vi "coler1.vi"(8 "error in":errorcluster, 11 "代刚":bool) -> (0 "error out":errorcluster, 1 "顏色":enum16{"黑色", "藍色", "綠色", "黃色", "紅色"}[](array[ring]))   [LabVIEW 2018]
uses:
  <vilib>/vision/NI_Vision_Development_Module.lvlib
panel:
  out "5":u32(colorbox)
  out "4":u32(colorbox)
  out "3":u32(colorbox)
  out "2":u32(colorbox)
  out "1":u32(colorbox)
  out "Color":u32(colorbox)
  out "亮度":dbl[](array[numeric])
  out "︹办":dbl[](array[numeric])
  out "Image Out":T1(plugin-control)
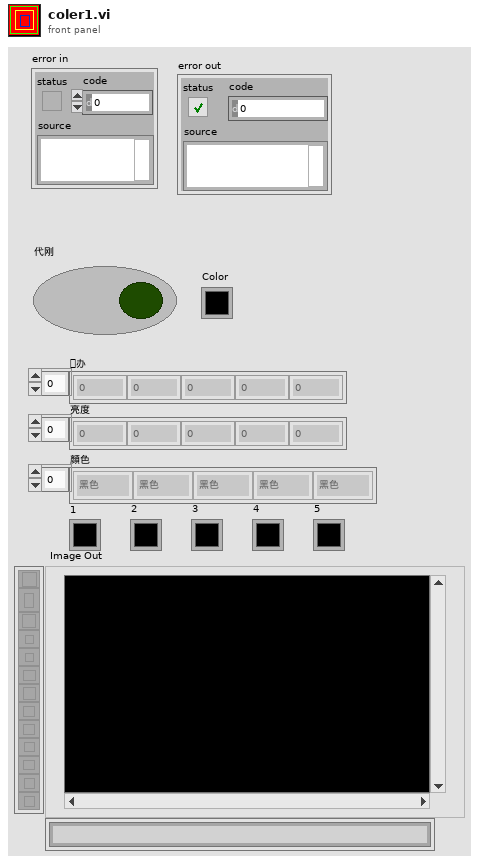
[diagram p1: front panel]
types:
  T1 = typedef "IMAQ Image.ctl" = refnum<image>
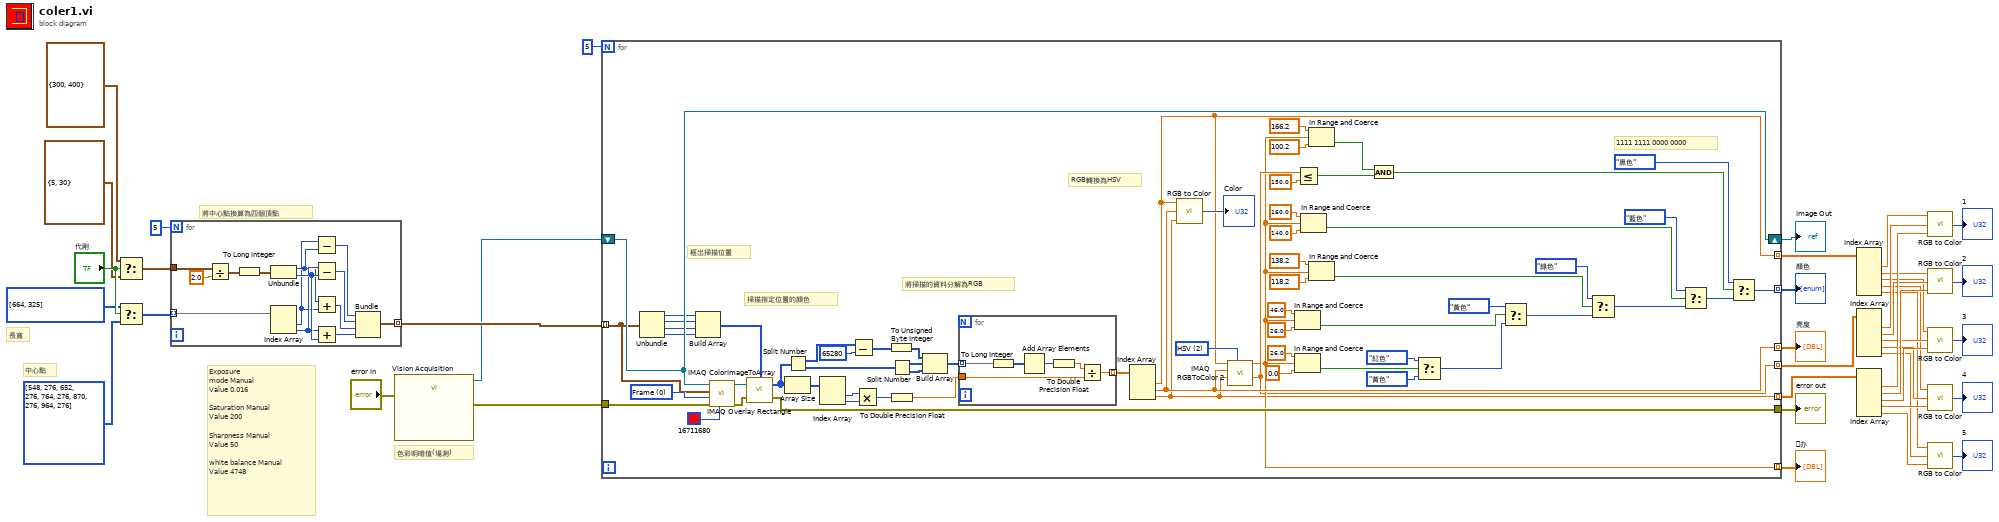
[diagram p0: block diagram]
diagram:
  # "長寬"
  # "Exposure\nmode Manual\nValue 0.016\n\nSaturation Manual\nValue 200\n\nSharpness Manual\nValue 50\n\nwhite balance Manual \nValue 4748"
  # "色彩明暗值(場測)"
  # "中心點"
  # "將中心點換算為四個頂點"
  n1 = Select(t=cluster{i32, i32} {300, 400}, s="代刚", f=cluster{i32, i32} {5, 30}) -> (s? t:f=w36:cluster{i32, i32})
  n2 = Select(t=i32[][] [[664, 325]], s="代刚", f=i32[][] [[548, 276], [652, 276], [764, 276], [870, 276], [964, 276]]) -> (s? t:f=w37:i32[][])
  n3 = for {
    N: 5 -> [_]
    tunnel: w36 -> [w55]
    tunnel: w37 -> [w52] mode=indexing
    tunnel: [w42] -> w38 mode=indexing
    n4 = Divide(x=w55, y=2.0) -> (x/y=w53:cluster{dbl, dbl})
    n5 = To Long Integer(number=w53) -> (32bit integer=w51:cluster{i32, i32})
    n6 = Unbundle(w51) -> (w48:i32, w50:i32)
    n7 = Index Array(array=w52) -> (element #1=w47:i32, element #2=w49:i32)  [unwired: 2 in]
    n8 = Subtract(x=w47, y=w48) -> (x-y=w46:i32)
    n9 = Subtract(x=w49, y=w50) -> (x-y=w45:i32)
    n10 = Add(x=w48, y=w47) -> (x+y=w44:i32)
    n11 = Add(x=w49, y=w50) -> (x+y=w43:i32)
    n12 = Bundle(w46, w45, w44, w43) -> (w42:cluster{i32, i32, i32, i32})  [unwired: 1 in]
  }
  n13 = call "Vision Acquisition"("error in"="error in") -> ("Image Out"=w33:T1, "error out"=w35:errorcluster)  [unwired: 25 in]
  n14 = for {
    N: 5 -> [_]
    shift-right: [w100] -> w34
    shift-left: w33 -> [w100]
    tunnel: w35 -> [w102]
    tunnel: [w101] -> w41
    tunnel: w38 -> [w96] mode=indexing
    tunnel: [w60] -> w26 mode=indexing
    tunnel: [w87] -> w25 mode=indexing
    tunnel: [w70] -> w24 mode=indexing
    tunnel: [w58] -> w23 mode=indexing
    tunnel: [w57] -> w22 mode=indexing
    tunnel: [w56] -> w21 mode=indexing
    w104 = u16 2 items=["RGB", "HSL", "HSV", "HSI", "CIE L*a*b*", "CIE XYZ"] ("Color Mode")
    w119 = u32 0 items=["Frame", "Fill", "Highlight"] ("Drawing Mode (Frame)")
    # "RGB轉換為HSV"
    # "將掃描的資料分解為RGB"
    # "掃描指定位置的顏色"
    # "框出掃描位置"
    # "1111 1111 0000 0000"
    n15 = Unbundle(w96) -> (w95:i32, w94:i32, w93:i32, w92:i32)
    n16 = Build Array(w95, w94, w93, w92) -> (w91:i32[])
    n17 = call "IMAQ Overlay Rectangle"("Color"=u32 16711680, "error in (no error)"=w102, "Drawing Mode (Frame)"=w119, "Rectangle"=w96, "Image"=w100) -> ("error out"=w98:errorcluster, "Image Out"=w99:T1)  [unwired: 5 in]
    n18 = call "IMAQ ColorImageToArray"("Optional Rectangle"=w91, "Image"=w99, "error in (no error)"=w98) -> ("Image Pixels (U32)"=w118:u32[][], "error out"=w101:errorcluster)  [unwired: 1 in, 1 out]
    n19 = Array Size(array=w118) -> (size(s)=w117:i32[])
    n20 = Split Number(x=w118) -> (hi(x)=w97:u16[][], lo(x)=w114:u16[][])
    n21 = Index Array(array=w117) -> (element #1=w108:i32, element #2=w109:i32)  [unwired: 2 in]
    n22 = Subtract(x=w97, y=u16 65280) -> (x-y=w115:u16[][])
    n23 = Multiply(x=w108, y=w109) -> (x*y=w107:i32)
    n24 = To Unsigned Byte Integer(number=w115) -> (unsigned 8bit integer=w113:u8[][])
    n25 = To Double Precision Float(number=w107) -> (double precision float=w106:dbl)
    n26 = Split Number(x=w114) -> (hi(x)=w112:u8[][], lo(x)=w111:u8[][])
    n27 = Build Array(w113, w112, w111) -> (w110:u8[][][])
    n28 = for {
      tunnel: w110 -> [w125] mode=indexing
      tunnel: w106 -> [w123]
      tunnel: [w122] -> w105 mode=indexing
      n29 = To Long Integer(number=w125) -> (32bit integer=w124:i32[][])
      n30 = Add Array Elements(numeric array=w124) -> (sum=w121:i32)
      n31 = To Double Precision Float(number=w121) -> (double precision float=w120:dbl)
      n32 = Divide(x=w120, y=w123) -> (x/y=w122:dbl)
    }
    n33 = Index Array(array=w105) -> (element #1=w58:dbl, element #2=w57:dbl, element #3=w56:dbl)  [unwired: 3 in]
    n34 = call <vilib>:"RGB to Color.vi"("B"=w56, "G"=w57, "R"=w58) -> ("Color"=→"Color":u32)
    n35 = call "IMAQ RGBToColor 2"("Color Mode"=w104, "Blue value"=w56, "Green value"=w57, "Red value"=w58) -> ("Blue or Luma or Val or Inten or Z or b*value"=w87:dbl, "Red or Hue or X or L* value"=w60:dbl)  [unwired: 4 in, 2 out]
    n36 = In Range and Coerce(upper limit=46.0, x=w60, lower limit=26.0) -> (In Range?=w72:bool)  [unwired: 1 out]
    n37 = In Range and Coerce(upper limit=26.0, x=w60, lower limit=0.0) -> (In Range?=w63:bool)  [unwired: 1 out]
    n38 = Less Or Equal?(x=w87, y=150.0) -> (x <= y?=w84:bool)
    n39 = In Range and Coerce(upper limit=160.0, x=w60, lower limit=140.0) -> (In Range?=w80:bool)  [unwired: 1 out]
    n40 = In Range and Coerce(upper limit=166.2, x=w60, lower limit=100.2) -> (In Range?=w85:bool)  [unwired: 1 out]
    n41 = In Range and Coerce(upper limit=138.2, x=w60, lower limit=118.2) -> (In Range?=w76:bool)  [unwired: 1 out]
    n42 = And(x=w85, y=w84) -> (x .and. y?=w83:bool)
    n43 = Select(t=enum16{"黑色", "藍色", "綠色", "黃色", "紅色"}."紅色", s=w63, f=enum16{"黑色", "藍色", "綠色", "黃色", "紅色"}."黃色") -> (s? t:f=w64:enum16{"黑色", "藍色", "綠色", "黃色", "紅色"})
    n44 = Select(t=enum16{"黑色", "藍色", "綠色", "黃色", "紅色"}."黃色", s=w72, f=w64) -> (s? t:f=w67:enum16{"黑色", "藍色", "綠色", "黃色", "紅色"})
    n45 = Select(t=enum16{"黑色", "藍色", "綠色", "黃色", "紅色"}."綠色", s=w76, f=w67) -> (s? t:f=w68:enum16{"黑色", "藍色", "綠色", "黃色", "紅色"})
    n46 = Select(t=enum16{"黑色", "藍色", "綠色", "黃色", "紅色"}."藍色", s=w80, f=w68) -> (s? t:f=w69:enum16{"黑色", "藍色", "綠色", "黃色", "紅色"})
    n47 = Select(t=enum16{"黑色", "藍色", "綠色", "黃色", "紅色"}."黑色", s=w83, f=w69) -> (s? t:f=w70:enum16{"黑色", "藍色", "綠色", "黃色", "紅色"})
  }
  "Image Out" <- w34
  "error out" <- w41
  "︹办" <- w26
  "亮度" <- w25
  "顏色" <- w24
  n48 = Index Array(array=w23) -> (element #1=w20:dbl, element #2=w17:dbl, element #3=w14:dbl, element #4=w11:dbl, element #5=w8:dbl)  [unwired: 5 in]
  n49 = Index Array(array=w22) -> (element #1=w19:dbl, element #2=w16:dbl, element #3=w13:dbl, element #4=w10:dbl, element #5=w7:dbl)  [unwired: 5 in]
  n50 = Index Array(array=w21) -> (element #1=w18:dbl, element #2=w15:dbl, element #3=w12:dbl, element #4=w9:dbl, element #5=w6:dbl)  [unwired: 5 in]
  n51 = call <vilib>:"RGB to Color.vi"("B"=w18, "G"=w19, "R"=w20) -> ("Color"=→"1":u32)
  n52 = call <vilib>:"RGB to Color.vi"("B"=w15, "G"=w16, "R"=w17) -> ("Color"=→"2":u32)
  n53 = call <vilib>:"RGB to Color.vi"("B"=w12, "G"=w13, "R"=w14) -> ("Color"=→"3":u32)
  n54 = call <vilib>:"RGB to Color.vi"("B"=w9, "G"=w10, "R"=w11) -> ("Color"=→"4":u32)
  n55 = call <vilib>:"RGB to Color.vi"("B"=w6, "G"=w7, "R"=w8) -> ("Color"=→"5":u32)
